vi "Write Device Identification.vi"(8 "error in":errorcluster, 10 "objects":T1[](array[typedef]) {"Object ID" format="%x"}, 11 "Modbus slave in":refnum<class "Modbus Slave.lvclass">) -> (0 "error out":errorcluster, 3 "Modbus slave out":refnum<class "Modbus Slave.lvclass">)   [LabVIEW 2012, in "Modbus Slave.lvclass"]
doc: "Writes Modbus object information stored on the device. This can include basic information, like manufacturer, additional standard items, or model-specific extended items. This function may take a large amount of time to execute, as it requires the transfer of a large quantity of binary data. Even on TCP/IP, this function is limited by the maximum defined size of a Modbus protocol data unit. If a slave supports objects, it is required that it stores information for VendorName (0x00), ProductCode (0x01), and MajorMinorRevision (0x02). The standard device data model provided by this library accepts any object request and can store any objects."
uses:
  Modbus Slave.lvclass
  Data Model/Identification Parameters.ctl
  Modbus Slave.lvclass/Modbus Slave.ctl
  Data Model/Device Data Model.lvclass
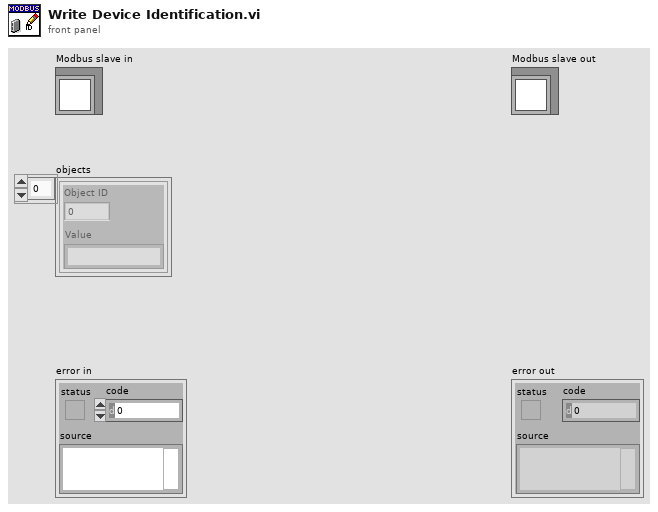
[diagram p1: front panel]
types:
  T1 = typedef "Device Data Model.lvclass/Identification Parameters.ctl" = cluster{"Object ID":u8, "Value":string}
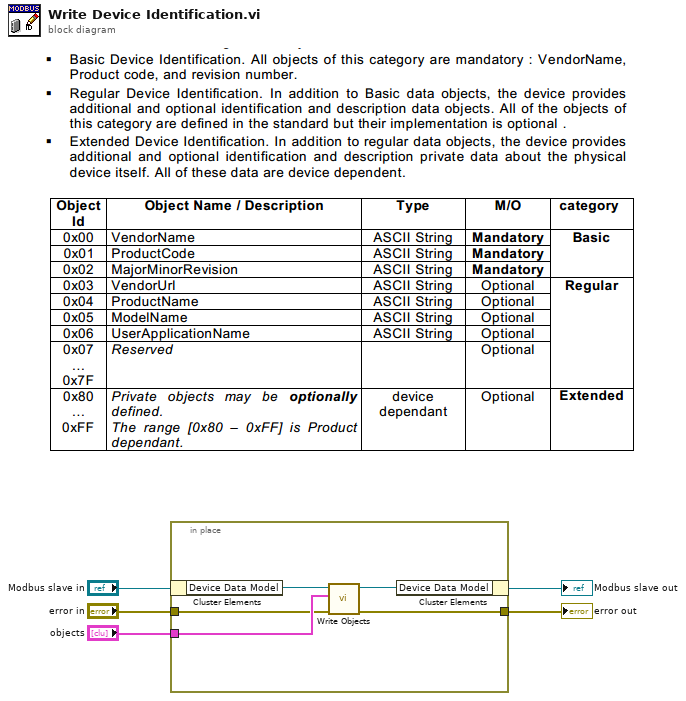
[diagram p0: block diagram]
diagram:
  n1 = in-place {
    in-place-border: [w10] -> w3
    in-place-border: "objects" -> [w9]
    in-place-border: "error in" -> [w7]
    n2 = in-place-cluster #1("Modbus slave in") -> ("Device Data Model"=w8:refnum<class "Device Data Model.lvclass">)
    n3 = call-dynamic "Write Objects.vi"("error in"=w7, "Objects"=w9, "device data model in"=w8) -> ("error out"=w10:errorcluster, "device data model out"=w6:refnum<class "Device Data Model.lvclass">)  [unwired: 7 in]
    n4 = in-place-cluster #1("Device Data Model"=w6) -> (→"Modbus slave out":refnum<class "Modbus Slave.lvclass">)
  }
  "error out" <- w3
